vi "Process Data.vi"(8 "error in":errorcluster, 11 "XML Editor GUI in":refnum<class "XML Editor GUI.lvclass">) -> (0 "error out":errorcluster, 3 "XML Editor GUI out":refnum<class "XML Editor GUI.lvclass">)   [LabVIEW 2014, in "XML Editor GUI.lvclass"]
uses:
  XML Editor GUI.lvclass
  Architecture/Classes/Topic_class/Topic.lvclass
  Controls/Custom Controls/Filter Buttons.ctl
  Controls/Filter Group.ctl
panel:
  out "Base?":bool
  in  "Matching Elements Listbox":i32(listbox)
  in  "Filter Group Array":T1[](array[typedef])
  in  "Attribute Name Filter Buttons":T2
  in  "Element Name Filter Buttons":T2
  in  "Attribute Value Filter Buttons":T2
  in  "Add Filter":bool
  in  "Attribute Value Listbox":i32(listbox)
  in  "Attribute Name Listbox":i32(listbox)
  in  "Element Name Listbox":i32(listbox)
  in  "Hide":bool
  in  "Attribute Value":string
  in  "Attribute Name":string
  in  "Element Name":string
  in  "Settings":bool
  in  "Load XML":bool
  in  "Tree":string(tree)
  # "All filters"
  # "Is this an element\nthe search started with?"
  # "Create views in configuration that is appropriate for each xml file type and task:\nie, Test Config changing limits to common subtests.\nThese views should just be a collection of filters with or without values in the filters"
  # "Allow for Regex"
  # "Number of Matching Elements"
  # "This should show the xml pretty print\nof the first line of each match, and line number"
  # "or"
  # "have matching element, Att Name and Att Value"
  # "Select rows to filter out common"
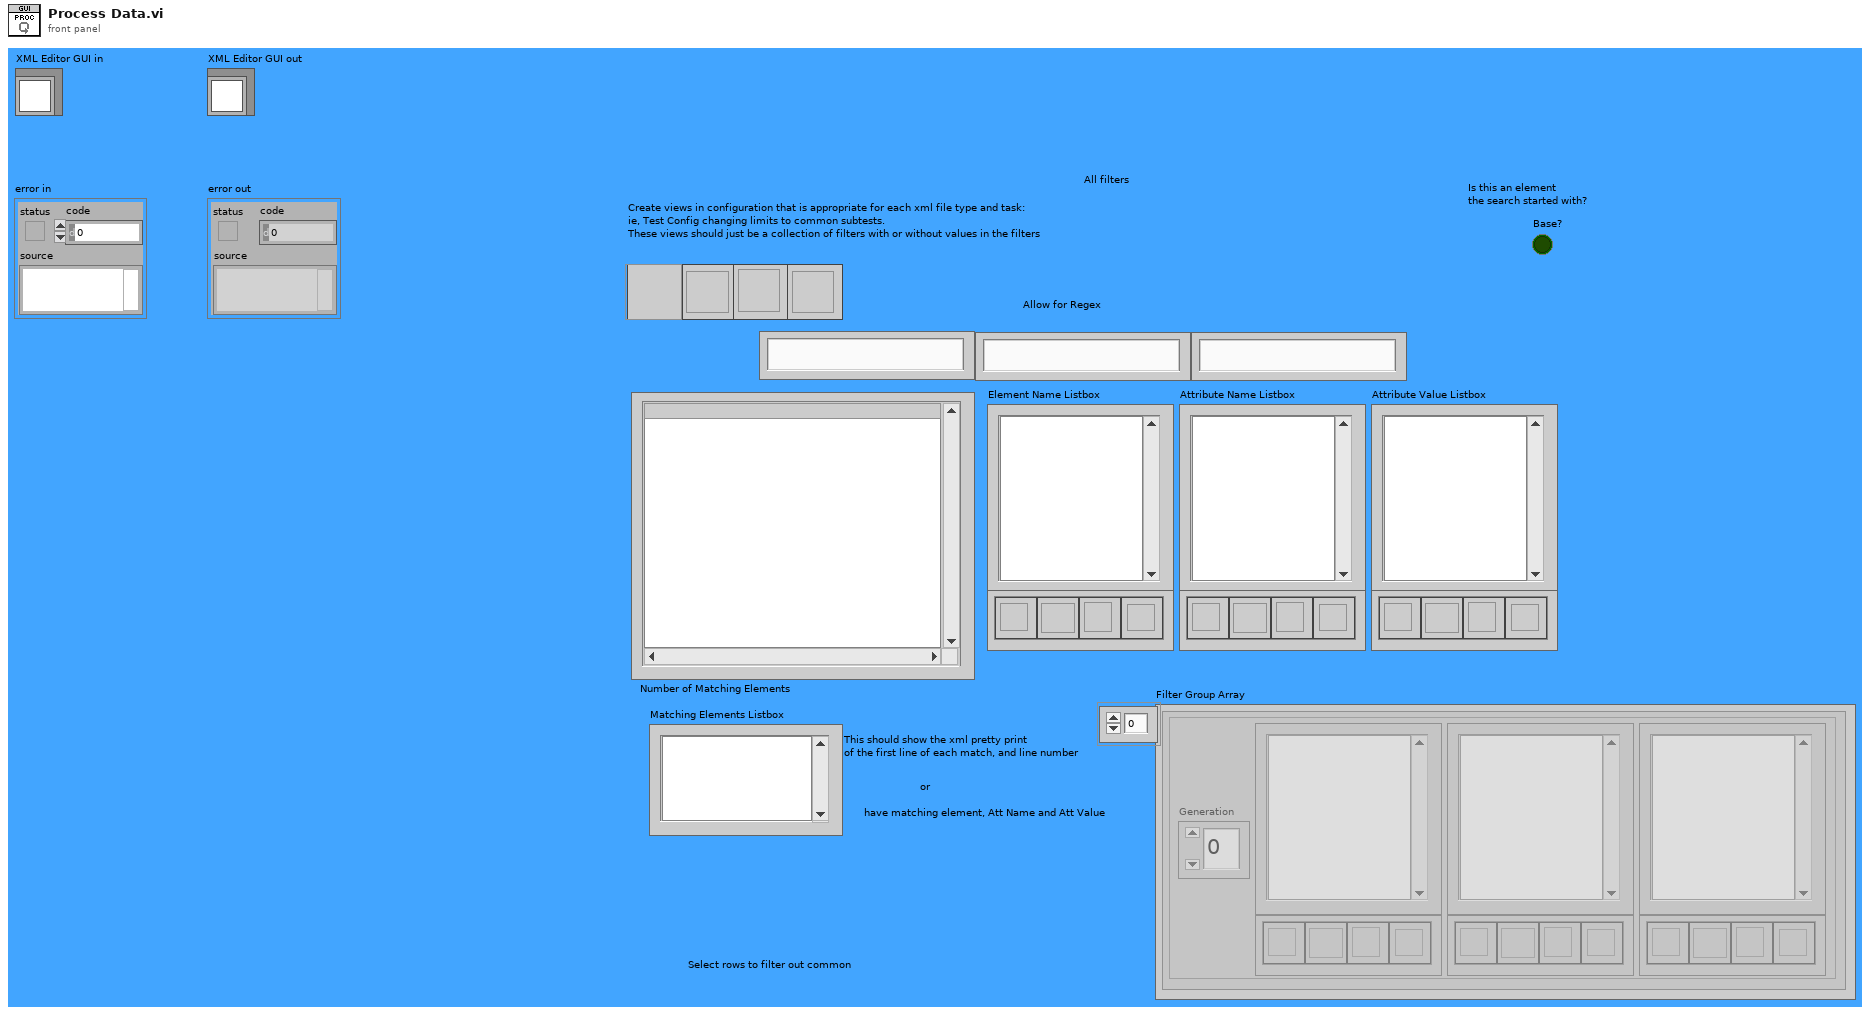
[diagram p1: front panel]
types:
  T1 = typedef "Filter Group.ctl" = cluster{"Generation":dbl, "Element Name Listbox":i32, "Attribute Name Listbox":i32, "Attribute Value Listbox":i32, "Attribute Value Filter Buttons":T2, "Element Name Filter Buttons":T2, "Attribute Name Filter Buttons":T2}
  T2 = typedef "Filter Buttons.ctl" = cluster{"Edit":bool, "Clear":bool, "Delete":bool, "Add":bool}
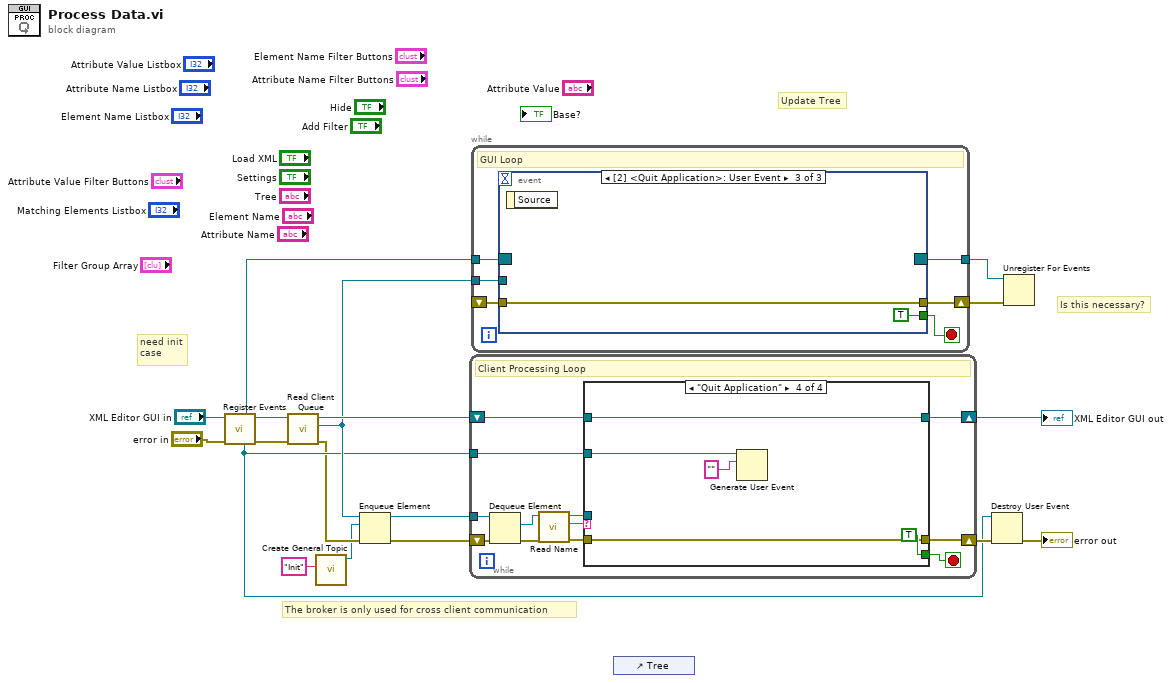
[diagram p0: block diagram]
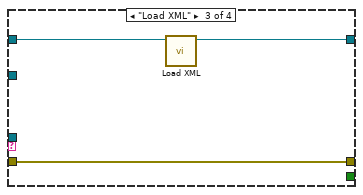
[diagram p4: hidden frame]
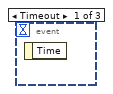
[diagram p5: hidden frame]
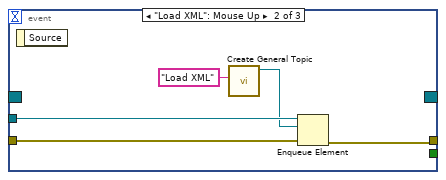
[diagram p6: hidden frame]
diagram:
  # "Update Tree"
  # "Is this necessary?"
  # "need init\ncase"
  # "The broker is only used for cross client communication"
  n1 = call "Register Events.vi"("error in"="error in", "XML Editor GUI in"="XML Editor GUI in") -> ("error out"=w6:errorcluster, "XML Editor GUI out"=w10:refnum<class "XML Editor GUI.lvclass">, "user event out"=w8:refnum<user-event>, "Event Registration Refnum"=w9:refnum<event-registration>)  [unwired: 6 in]
  n2 = call-dynamic "Read Client Queue.vi"("error in"=w6, "Client in"=w10) -> ("error out"=w3:errorcluster, "Client Queue"=w13:refnum<queue>, "Client out"=w17:refnum<class "XML Editor GUI.lvclass">)  [unwired: 7 in]
  n3 = call "Create General Topic.vi"("Name"="Init") -> ("Topic out"=w1:refnum<class "Topic.lvclass">)  [unwired: 9 in, 1 out]
  n4 = Enqueue Element(queue=w13, element=w1, error in (no error)=w3) -> (queue out=w4:refnum<queue>, error out=w2:errorcluster)  [unwired: 1 in, 1 out]
  n5 = while {
    tunnel: w4 -> [w28]
    shift-right: [w22] -> w18
    shift-left: w2 -> [w25]
    tunnel: w8 -> [w21]
    shift-right: [w19] -> w15
    shift-left: w17 -> [w20]
    stop <- w24 stop-if-true
    # "Client Processing Loop"
    n6 = Dequeue Element(queue=w28, error in (no error)=w25) -> (element=w29:refnum<class "Topic.lvclass">, error out=w30:errorcluster)  [unwired: 1 in, 2 out]
    n7 = call-dynamic "Read Name.vi"("error in"=w30, "Topic in"=w29) -> ("error out"=w23:errorcluster, "Name"=w27:string, "Topic out"=w26:refnum<class "Topic.lvclass">)  [unwired: 7 in]
    n8 = case shown="\"Quit Application\"" w27 {
      tunnel: w26 -> [_ _ _ _]
      tunnel: [_ _ _ TRUE] -> w24
      tunnel: w23 -> [w32 _ w36 w40]
      tunnel: [w32 _ w36 w40] -> w22
      tunnel: w21 -> [_ _ _ w38]
      tunnel: w20 -> [w31 w33 w35 w37]
      tunnel: [w31 w33 w34 w37] -> w19
      frame Default {
      }
      frame "Init" {
      }
      frame "Load XML" {
        n9 = call "Load XML.vi"("XML Editor GUI in"=w35) -> ("XML Editor GUI out"=w34:refnum<class "XML Editor GUI.lvclass">)  [unwired: 9 in, 1 out]
      }
      frame "Quit Application" {
        n10 = Generate User Event(user event=w38, event data cluster="" ("event data")) -> ()  [unwired: 2 in, 2 out]
      }
    }
  }
  "XML Editor GUI out" <- w15
  n11 = while {
    shift-right: [w45] -> w11
    shift-left: _ -> [w46]
    tunnel: w13 -> [w44]
    tunnel: [w43] -> w12
    tunnel: w9 -> [w42]
    stop <- w47 stop-if-true
    # "GUI Loop"
    n12 = event shown="[2] <Quit Application>: User Event" {
      selector: w42 -> [_ _ _]
      dyn-events: [_ _ _] -> w43
      timeout: _ -> [_ _ _]
      tunnel: [_ _ TRUE] -> w47
      tunnel: w46 -> [_ w52 w53]
      tunnel: [_ w51 w53] -> w45
      tunnel: w44 -> [_ w50 _]
      event Timeout {
        n13 = event-data() -> ()  [unwired: 1 in, 1 out]
      }
      event "Load XML": Mouse Up {
        n14 = event-data() -> ()  [unwired: 1 in, 1 out]
        n15 = call "Create General Topic.vi"("Name"="Load XML") -> ("Topic out"=w49:refnum<class "Topic.lvclass">)  [unwired: 9 in, 1 out]
        n16 = Enqueue Element(queue=w50, element=w49, error in (no error)=w52) -> (error out=w51:errorcluster)  [unwired: 1 in, 2 out]
      }
      event User Event {
        n17 = event-data() -> ()  [unwired: 1 in, 1 out]
      }
    }
  }
  n18 = control-ref of="Tree"() -> ()  [unwired: 1 out]
  n19 = Destroy User Event(user event=w8, error in=w18) -> (error out=→"error out":errorcluster)
  n20 = Unregister For Events(event registration refnum=w12, error in=w11) -> ()  [unwired: 1 out]
